vi "Windows Simulate 4 Wire xVDT.vi"() -> ()   [LabVIEW 2011]
panel:
  in  "Stimulus Volts":i16=13
  out "LVDT":dynamicdata(graph)
  in  "Position (mm)":dbl(slide) caption="Position" scale=-20.0..20.0 scale format="%.2f"
  in  "Sensitivity (V/V/mm)":dbl=0.05
  in  "stop":bool
  in  "Scaling Factor":fxp<+/-,19,5>
  # "Setup"
  # "Run-Time"
  # "Display"
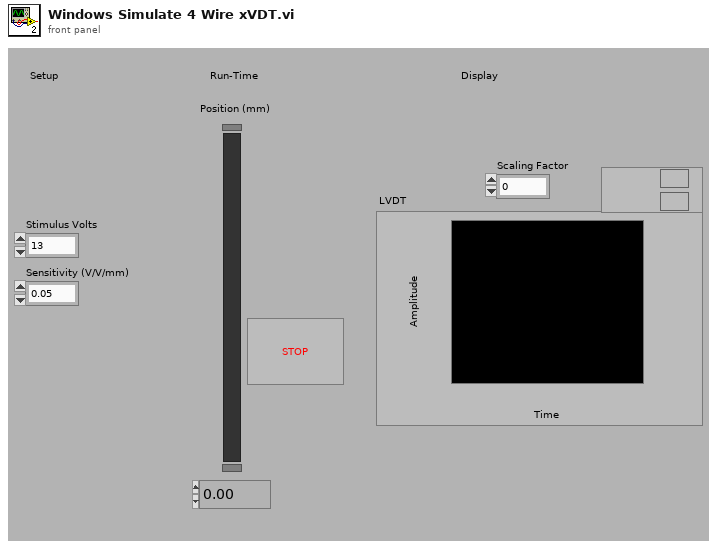
[diagram p1: front panel]
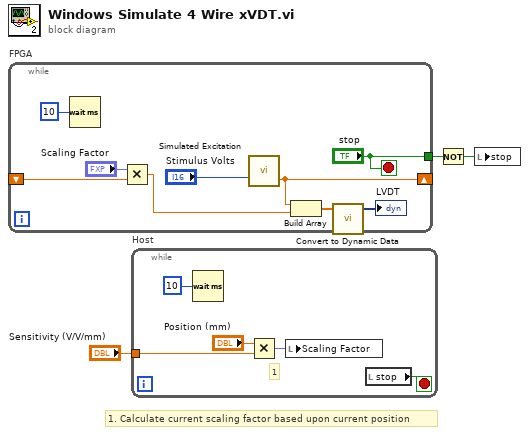
[diagram p0: block diagram]
diagram:
  # "1. Calculate current scaling factor based upon current position"
  n1 = while "FPGA" {
    shift-right: [w7] -> _
    shift-left: _ -> [w6]
    tunnel: ["stop"] -> w3
    stop <- "stop" stop-if-true
    n2 = Wait (ms)(milliseconds to wait=u32 10) -> ()  [unwired: 1 out]
    n3 = Multiply(x="Scaling Factor", y=w6) -> (x*y=w5:dbl)
    n4 = call "Simulated Excitation.vi"("Volts"="Stimulus Volts") -> ("Analog Input"=w7:dbl)  [unwired: 2 in]
    n5 = Build Array(w7, w5) -> (w10:dbl[])
    n6 = call "Convert to Dynamic Data"("Array"=w10) -> ("Dynamic Data Type"=→"LVDT":dynamicdata)  [unwired: 3 in]
  }
  n7 = while "Host" {
    tunnel: "Sensitivity (V/V/mm)" -> [w14]
    stop <- w17 stop-if-true
    # "1"
    n8 = Wait (ms)(milliseconds to wait=u32 10) -> ()  [unwired: 1 out]
    n9 = Multiply(x="Position (mm)", y=w14) -> (x*y=w13:fxp<+/-,19,5>)
    n10 = local write "Scaling Factor"(w13) -> ()
    n11 = local read "stop"() -> (w17:bool)
  }
  n12 = Not(x=w3) -> (.not. x?=w2:bool)
  n13 = local write "stop"(w2) -> ()
